vi "testPersistentData.vi"() -> ()   [LabVIEW 2019, in "TestCaseTest.lvlib" / "Theory.lvlib"]
uses:
  Theory.lvlib
  TestCase/Theory/Theory.lvclass
  TestCaseTestSupport/FakeTheory.vi
  TestCaseTestSupport/TestCaseTestSupport.lvlib
  Assertion/Assertion.lvlib
panel:
  out "error out":errorcluster
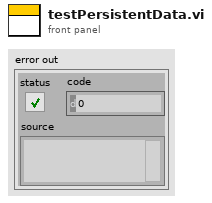
[diagram p1: front panel]
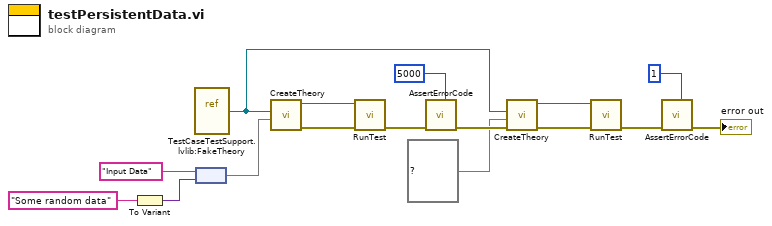
[diagram p0: block diagram]
diagram:
  n1 = To Variant(anything="Some random data" ("key")) -> (Variant=w10:variant)
  n2 = vi-ref "TestCaseTestSupport.lvlib:FakeTheory.vi"() -> (w1:refnum<vi>)
  n3 = node("Input Data" ("key"), w10) -> (w11:map{string, variant})
  n4 = call "CreateTheory.vi"("Control Data"=w11, "VI Refnum"=w1) -> ("error out"=w15:errorcluster, "Theory"=w16:refnum<class "Theory.lvclass">)  [unwired: 8 in]
  n5 = call-dynamic "RunTest.vi"("error in (no error)"=w15, "Theory in"=w16) -> ("error out"=w14:errorcluster)  [unwired: 8 in, 1 out]
  n6 = call "AssertErrorCode.vi"("Expected"=5000, "error in (no error)"=w14) -> ("error out"=w6:errorcluster)  [unwired: 9 in]
  n7 = call "CreateTheory.vi"("error in (no error)"=w6, "Control Data"=map{string, variant} {}, "VI Refnum"=w1) -> ("error out"=w8:errorcluster, "Theory"=w7:refnum<class "Theory.lvclass">)  [unwired: 7 in]
  n8 = call-dynamic "RunTest.vi"("error in (no error)"=w8, "Theory in"=w7) -> ("error out"=w5:errorcluster)  [unwired: 8 in, 1 out]
  n9 = call "AssertErrorCode.vi"("Expected"=1, "error in (no error)"=w5) -> ("error out"=→"error out":errorcluster)  [unwired: 9 in]
